vi "YKMW100 Mode Control.vi"(0 "VISA session":refnum<visa-resource-name>="MW100", 5 "Model":enum16{"Meausurement Mode", "Setting Mode"}(ring), 11 "error in (no error)":errorcluster) -> (4 "dup VISA session":refnum<visa-resource-name>="MW100", 15 "error out":errorcluster)   [LabVIEW 2009]
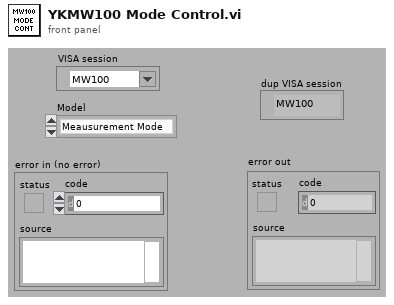
[diagram p1: front panel]
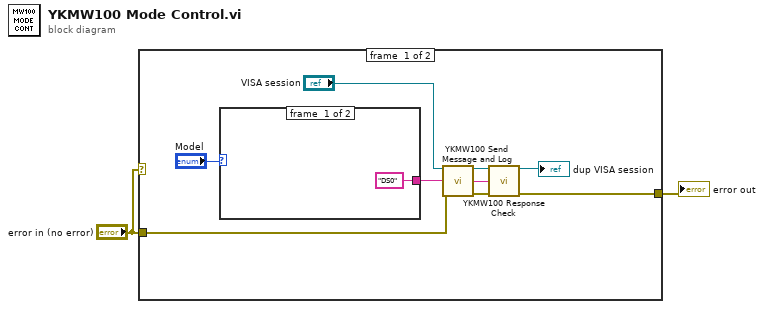
[diagram p0: block diagram]
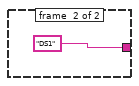
[diagram p2: hidden frame]
diagram:
  n1 = case shown="Error" "error in (no error)" {
    selector: "error in (no error)" -> [_ w14]
    tunnel: [w7 w14] -> w2
    tunnel: "error in (no error)" -> [w3 _]
    frame #0 {
      n2 = case shown="\"Meausurement Mode\", Default" "Model" {
        tunnel: ["DS0" ("Send Message (\"\")") "DS1" ("Send Message (\"\")")] -> w5
        frame #0 {
        }
        frame #1 {
        }
      }
      n3 = call "YKMW100 Send Message and Log.vi"("VISA session"="VISA session", "Send Message (\"\")"=w5, "error in (no error)"=w3) -> ("dup VISA session"=w11:refnum<visa-resource-name>, "Read Buffer"=w9:string, "error out"=w10:errorcluster)  [unwired: 10 in]
      n4 = call "YKMW100 Response Check.vi"("VISA session"=w11, "Message In (\"\")"=w9, "error in (no error)"=w10) -> ("dup VISA session"=→"dup VISA session":refnum<visa-resource-name>, "error out"=w7:errorcluster)  [unwired: 8 in, 3 out]
    }
    frame #1 {
    }
  }
  "error out" <- w2
